vi "Acquire Two Temperature Calibration Points.vi"() -> ()   [LabVIEW 2018]
doc: "Paul Packebush"
uses:
  Global.gbl
  Use Software Adjust on Measurements.vi/AI Read (scaled array).vi
  <vilib>/Analysis/NI_AALBase.lvlib
  <vilib>/Analysis/baseanly.llb/Mean (DBL).vi
panel:
  out "mean":dbl format="%.5f"
  out "Second Point":dbl(graph)=49.91505165100098
  in  "Second Point\n(Deg C)":dbl=50.0 format="%.2f"
  in  "First Point\n(Deg C)":dbl format="%.2f"
  out "mean":dbl format="%.5f"
  out "First Point":dbl(graph)=-0.10996673010289669
  in  "number of scans to acquire":i32=100
  in  "scan rate":sgl=1000.0 format="%.2f"
  in  "channels":string[](array[string])=["temp"]
  in  "device":i16=1
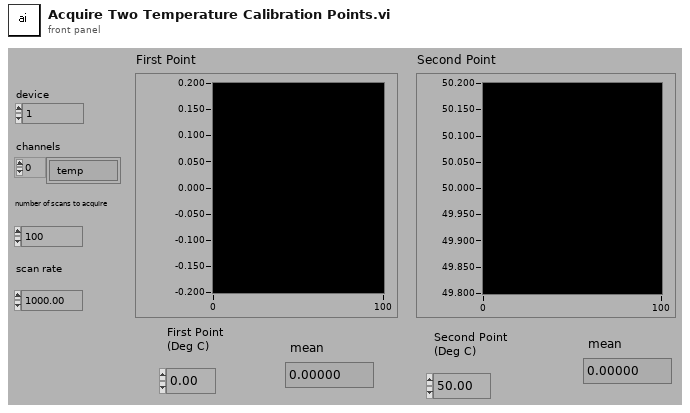
[diagram p1: front panel]
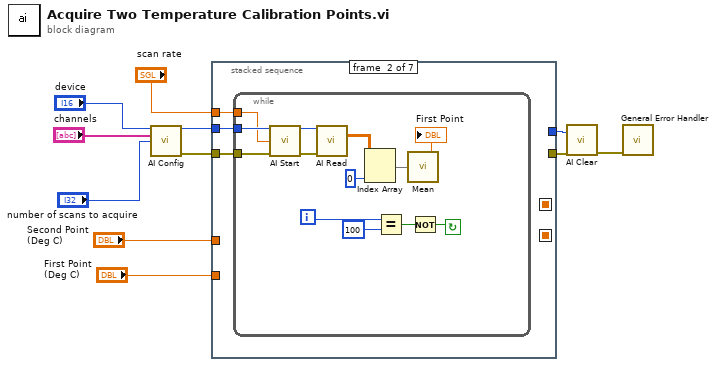
[diagram p0: block diagram]
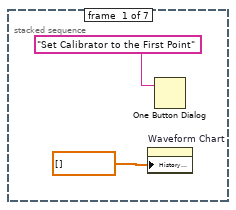
[diagram p2: hidden frame]
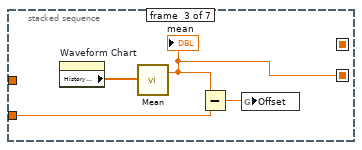
[diagram p3: hidden frame]
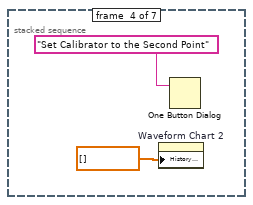
[diagram p4: hidden frame]
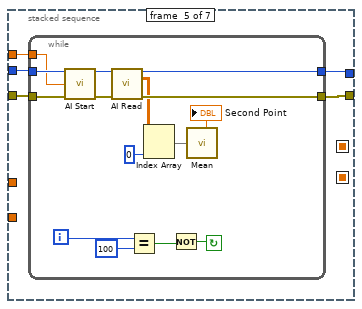
[diagram p5: hidden frame]
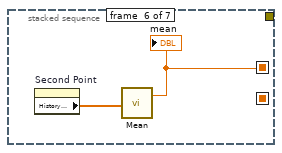
[diagram p6: hidden frame]
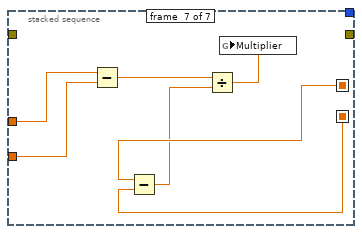
[diagram p7: hidden frame]
diagram:
  n1 = call "AI Config.vi"("device (1)"="device", "channels (0)"="channels", "buffer size (1000 scans)"="number of scans to acquire") -> ("taskID"=w8:u32, "error out"=w11:errorcluster)  [unwired: 10 in, 1 out]
  n2 = stacked-sequence {
    seq-local: [_ _ w30 _ _ _ _] -> [_ _ _ _ _ _ w61]
    seq-local: [_ _ _ _ _ w56 _] -> [_ _ _ _ _ _ w60]
    tunnel: w11 -> [_ w16 _ _ w39 _ _]
    tunnel: [_ _ _ _ w38 _ _] -> w4
    tunnel: w8 -> [_ w15 _ _ w40 _ _]
    tunnel: [_ _ _ _ w37 _ _] -> w5
    tunnel: "First Point\n(Deg C)" -> [_ _ w32 _ _ _ w62]
    tunnel: "Second Point\n(Deg C)" -> [_ _ _ _ _ _ w63]
    tunnel: "scan rate" -> [_ w14 _ _ w36 _ _]
    frame #0 {
      n3 = property on="Waveform Chart" class="WFChart (strict)"("History Data"=dbl[] [] ("Write Attribute")) -> ()  [unwired: 2 in, 2 out]
      n4 = One Button Dialog(message="Set Calibrator to the First Point") -> ()  [unwired: 1 in, 1 out]
    }
    frame #1 {
      n5 = while {
        tunnel: w14 -> [w18]
        tunnel: w15 -> [w27]
        tunnel: w16 -> [w28]
        i -> [w20]
        stop <- w23 continue-if-true
        n6 = call "AI Start.vi"("taskID in"=w27, "scan rate (1000 scans/sec)"=w18, "error in (no error)"=w28) -> ("taskID out"=w26:u32, "error out"=w29:errorcluster)  [unwired: 9 in, 2 out]
        n7 = call-poly "AI Read.vi"("taskID in"=w26, "error in (no error)"=w29) -> ("scaled data"=w25:sgl[][])  [unwired: 8 in, 5 out]
        n8 = Index Array(array=w25, index (col)=0 ("Index")) -> (element=w22:sgl[])  [unwired: 1 in]
        n9 = Equal?(x=w20, y=100) -> (x = y?=w17:bool)
        n10 = call-poly <vilib>:"Mean.vi"("X"=w22) -> ("mean"=→"First Point":dbl)  [unwired: 1 out]
        n11 = Not(x=w17) -> (.not. x?=w23:bool)
      }
    }
    frame #2 {
      n12 = property on="Waveform Chart" class="WFChart (strict)"() -> ("History Data"=w33:dbl[])  [unwired: 2 in, 2 out]
      n13 = call-poly <vilib>:"Mean.vi"("X"=w33) -> ("mean"=w30:dbl)  [unwired: 1 out]
      "mean" <- w30
      n14 = Subtract(x=w30, y=w32) -> (x-y=w31:dbl)
      n15 = global write "Global.gbl" "Offset"(w31) -> ()
    }
    frame #3 {
      n16 = property on="Waveform Chart 2" class="WFChart (strict)"("History Data"=dbl[] [] ("Write Attribute")) -> ()  [unwired: 2 in, 2 out]
      n17 = One Button Dialog(message="Set Calibrator to the Second Point") -> ()  [unwired: 1 in, 1 out]
    }
    frame #4 {
      n18 = while {
        tunnel: w36 -> [w43]
        tunnel: [w50] -> w37
        tunnel: w40 -> [w52]
        tunnel: [w53] -> w38
        tunnel: w39 -> [w54]
        i -> [w45]
        stop <- w47 continue-if-true
        n19 = call "AI Start.vi"("taskID in"=w52, "scan rate (1000 scans/sec)"=w43, "error in (no error)"=w54) -> ("taskID out"=w51:u32, "error out"=w55:errorcluster)  [unwired: 9 in, 2 out]
        n20 = call-poly "AI Read.vi"("taskID in"=w51, "error in (no error)"=w55) -> ("taskID out"=w53:u32, "scaled data"=w49:sgl[][], "error out"=w50:errorcluster)  [unwired: 8 in, 3 out]
        n21 = Equal?(x=w45, y=100) -> (x = y?=w42:bool)
        n22 = Index Array(array=w49, index (col)=0 ("Index")) -> (element=w46:sgl[])  [unwired: 1 in]
        n23 = Not(x=w42) -> (.not. x?=w47:bool)
        n24 = call-poly <vilib>:"Mean.vi"("X"=w46) -> ("mean"=→"Second Point":dbl)  [unwired: 1 out]
      }
    }
    frame #5 {
      n25 = property on="Second Point" class="WFChart (strict)"() -> ("History Data"=w57:dbl[])  [unwired: 2 in, 2 out]
      n26 = call-poly <vilib>:"Mean.vi"("X"=w57) -> ("mean"=w56:dbl)  [unwired: 1 out]
      "mean" <- w56
    }
    frame #6 {
      n27 = Subtract(x=w63, y=w62) -> (x-y=w59:dbl)
      n28 = Subtract(x=w60, y=w61) -> (x-y=w58:dbl)
      n29 = Divide(x=w59, y=w58) -> (x/y=w64:dbl)
      n30 = global write "Global.gbl" "Multiplier"(w64) -> ()
    }
  }
  n31 = call "AI Clear.vi"("error in (no error)"=w5, "taskID in"=w4) -> ("error out"=w7:errorcluster)  [unwired: 4 in, 1 out]
  n32 = call <vilib>:"General Error Handler.vi"("error in (no error)"=w7) -> ()  [unwired: 10 in, 5 out]
